vi "PCAN_InitializeSession.vi"(8 "error in (no error)":errorcluster, 10 "TPCANBaudrate":T1, 11 "TPCANHandle":T2) -> (0 "error out":errorcluster)   [LabVIEW 2021, in "PCAN Reader.lvlib"]
uses:
  <instrlib>/KDI Digital Instrumentation/API_for_PCAN_BASIC_FD/TPCANHandle.ctl
  <instrlib>/KDI Digital Instrumentation/API_for_PCAN_BASIC_FD/TPCANBaudrate.ctl
  <instrlib>/KDI Digital Instrumentation/API_for_PCAN_BASIC_FD/TPCANParameter.ctl
  <instrlib>/KDI Digital Instrumentation/API_for_PCAN_BASIC_FD/Error language selector.ctl
  <instrlib>/KDI Digital Instrumentation/API_for_PCAN_BASIC_FD/PCAN Bus Off Auto Reset.ctl
  <instrlib>/KDI Digital Instrumentation/API_for_PCAN_BASIC_FD/PCAN Get CHANNEL CONDITION.vi
  PCAN Reader.lvlib
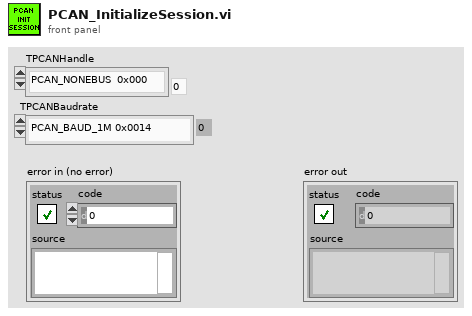
[diagram p1: front panel]
types:
  T1 = typedef "TPCANBaudrate.ctl" = enum16{"PCAN_BAUD_1M 0x0014", "PCAN_BAUD_800K 0x0016", "PCAN_BAUD_500K 0x001C", "PCAN_BAUD_250K 0x011C", "PCAN_BAUD_125K 0x031C", "PCAN_BAUD_100K 0x432F", "PCAN_BAUD_95K 0xC34E", "PCAN_BAUD_83K 0x852B", "PCAN_BAUD_50K 0x472F", "PCAN_BAUD_47K 0x1414", "PCAN_BAUD_33K 0x8B2F", "PCAN_BAUD_20K 0x532F", "PCAN_BAUD_10K 0x672F", "PCAN_BAUD_5K 0x7F7F", "User Baudrate"}
  T2 = typedef "TPCANHandle.ctl" = enum16{"PCAN_NONEBUS  0x000", "PCAN_ISABUS1  0x21", "PCAN_ISABUS2  0x22", "PCAN_ISABUS3  0x23", "PCAN_ISABUS4  0x24", "PCAN_ISABUS5  0x25", "PCAN_ISABUS6  0x26", "PCAN_ISABUS7  0x27", "PCAN_ISABUS8  0x28", "PCAN_DNGBUS1  0x31", "PCAN_PCIBUS1  0x41", "PCAN_PCIBUS1  0x42", "PCAN_PCIBUS1  0x43", "PCAN_PCIBUS1  0x44", "PCAN_PCIBUS1  0x45", "PCAN_PCIBUS1  0x46", "PCAN_PCIBUS1  0x47", "PCAN_PCIBUS1  0x48", "PCAN_PCIBUS1  0x409", "PCAN_PCIBUS1  0x40A", "PCAN_PCIBUS1  0x40B", "PCAN_PCIBUS1  0x40C", "PCAN_PCIBUS1  0x40D", "PCAN_PCIBUS1  0x40E", "PCAN_PCIBUS1  0x40F", "PCAN_PCIBUS1  0x410", "PCAN_USBBUS1  0x51", "PCAN_USBBUS2  0x52", "PCAN_USBBUS3  0x53", "PCAN_USBBUS4  0x54", "PCAN_USBBUS5  0x55", "PCAN_USBBUS6  0x56", "PCAN_USBBUS7  0x57", "PCAN_USBBUS8  0x58", "PCAN_USBBUS9  0x509", "PCAN_USBBUS10  0x50A", "PCAN_USBBUS11  0x50B", "PCAN_USBBUS12  0x50C", "PCAN_USBBUS13  0x50D", "PCAN_USBBUS14  0x50E", "PCAN_USBBUS15  0x50F", "PCAN_USBBUS16  0x510", "PCAN_PCCBUS1  0x61", "PCAN_PCCBUS2  0x62", "PCAN_LANBUS1  0x801", "PCAN_LANBUS2  0x802", "PCAN_LANBUS3  0x803", "PCAN_LANBUS4  0x804", "PCAN_LANBUS5  0x805", "PCAN_LANBUS6  0x806", "PCAN_LANBUS7  0x807", "PCAN_LANBUS8  0x808", "PCAN_LANBUS9  0x809", "PCAN_LANBUS10  0x80A", "PCAN_LANBUS11  0x80B", "PCAN_LANBUS12  0x80C", "PCAN_LANBUS13  0x80D", "PCAN_LANBUS14  0x80E", "PCAN_LANBUS15  0x80F", "PCAN_LANBUS16  0x810"}
  T3 = typedef "PCAN Bus Off Auto Reset.ctl" = enum32{"PCAN_PARAMETER_OFF", "PCAN_PARAMETER_ON"}
  T4 = typedef "TPCANParameter.ctl" = enum8{"Not Available", "PCAN device number", "PCAN 5-volt power", "PCAN receive event", "PCAN message filter", "PCAN API version", "PCAN channel version", "PCAN busoff autoreset", "PCAN listen-only", "PCAN log location", "PCAN log status", "PCAN log configure", "PCAN log text", "PCAN channel condition", "PCAN hardware name", "PCAN_RECEIVE_STATUS", "PCAN_CONTROLLER_NUMBER", "PCAN_TRACE_LOCATION ", "PCAN_TRACE_STATUS", "PCAN_TRACE_SIZE", "PCAN_TRACE_CONFIGURE", "PCAN_CHANNEL_IDENTIFYING", "PCAN_CHANNEL_FEATURES", "PCAN_SPEED_ADAPTING", "PCAN_BITRATE_INFO", "PCAN_BITRATE_INFO_FD", "PCAN_BUSSPEED_NOMINAL", "PCAN_BUSSPEED_DATA", "PCAN_IP_ADDRESS", "PCAN_LAN_SERVICE_STATUS", "PCAN_ALLOW_STATUS_FRAMES", "PCAN_ALLOW_RTR_FRAMES", "PCAN_ALLOW_ERROR_FRAMES", "PCAN_INTERFRAME_DELAY", "PCAN_ACCEPTANCE_FILTER_11BIT", "PCAN_ACCEPTANCE_FILTER_29BIT", "PCAN_IO_DIGITAL_CONFIGURATION", "PCAN_IO_DIGITAL_VALUE", "PCAN_IO_DIGITAL_SET", "PCAN_IO_DIGITAL_CLEAR", "PCAN_IO_ANALOG_VALUE", "PCAN_FIMRWARE_VRSION", "PCAN__ATTACHED_CHANNELS_COUNT", "PCAN_ATTACHED CHANNELS"}
  T5 = typedef "Error language selector.ctl" = u16
  T6 = typedef "Channel Availability.ctl" = enum16{"PCAN_CHANNEL_UNAVAILABLE", "PCAN_CHANNEL_AVAILABLE", "PCAN_CHANNEL_OCCUPIED", "PCAN_CHANNEL_PCANVIEW "}
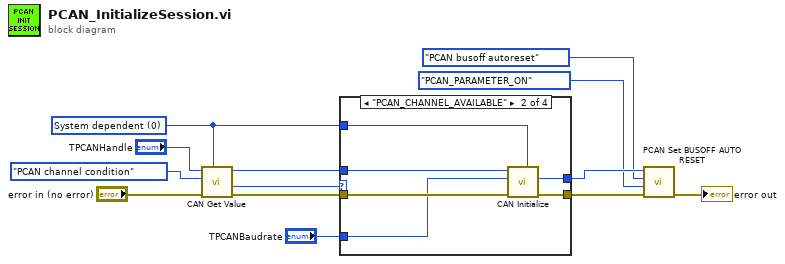
[diagram p0: block diagram]
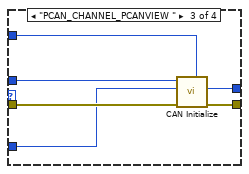
[diagram p3: hidden frame]
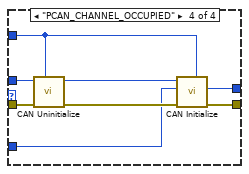
[diagram p4: hidden frame]
diagram:
  w7 = T5 0 items=["System dependent", "Not available", "Not available", "Not available", "Not available", "Not available", "Not available", "Deutsch", "Not available", "English", "Español", "Not available", "Français", "Not available", "Not available", "Not available", "Italiano"] ("Language")
  n1 = call-poly <instrlib>:"CAN Get Value.vi"("Language"=w7, "error in (no error)"="error in (no error)", "TPCANParameter"=TPCANParameter."PCAN channel condition", "TPCANHandle"="TPCANHandle") -> ("error out"=w10:errorcluster, "Channel condition"=w9:T6, "TPCANHandle out"=w8:T2)  [unwired: 5 in]
  n2 = case shown="\"PCAN_CHANNEL_AVAILABLE\"" w9 {
    tunnel: [w15 w21 w27 w35] -> w5
    tunnel: w7 -> [_ w20 w26 w32]
    tunnel: w10 -> [w15 w18 w24 w34]
    tunnel: w8 -> [w14 w19 w25 w33]
    tunnel: "TPCANBaudrate" -> [_ w17 w23 w29]
    tunnel: [w14 w16 w22 w28] -> w4
    frame "PCAN_CHANNEL_UNAVAILABLE", Default {
    }
    frame "PCAN_CHANNEL_AVAILABLE" {
      n3 = call <instrlib>:"CAN Initialize.vi"("Language"=w20, "error in (no error)"=w18, "TPCANBaudrate"=w17, "TPCANHandle"=w19) -> ("error out"=w21:errorcluster, "TPCANHandle_out"=w16:T2)  [unwired: 5 in, 1 out]
    }
    frame "PCAN_CHANNEL_PCANVIEW " {
      n4 = call <instrlib>:"CAN Initialize.vi"("Language"=w26, "error in (no error)"=w24, "TPCANBaudrate"=w23, "TPCANHandle"=w25) -> ("error out"=w27:errorcluster, "TPCANHandle_out"=w22:T2)  [unwired: 5 in, 1 out]
    }
    frame "PCAN_CHANNEL_OCCUPIED" {
      n5 = call <instrlib>:"CAN Uninitialize.vi"("Language"=w32, "error in (no error)"=w34, "TPCANHandle"=w33) -> ("error out"=w30:errorcluster, "TPCANHandle out"=w31:T2)  [unwired: 6 in, 1 out]
      n6 = call <instrlib>:"CAN Initialize.vi"("Language"=w32, "error in (no error)"=w30, "TPCANBaudrate"=w29, "TPCANHandle"=w31) -> ("error out"=w35:errorcluster, "TPCANHandle_out"=w28:T2)  [unwired: 5 in, 1 out]
    }
  }
  n7 = call <instrlib>:"PCAN Set BUSOFF AUTO RESET.vi"("error in (no error)"=w5, "BusOFF Auto Reset ON or OFF"=PCAN_Bus_Off_Auto_Reset."PCAN_PARAMETER_ON", "TPCANParameter"=TPCANParameter."PCAN busoff autoreset", "TPCANHandle"=w4) -> ("error out"=→"error out":errorcluster)  [unwired: 6 in, 1 out]
